vi "Read Exit Slit.vi"(8 "error in (no error)":errorcluster, 11 "Spectrometer Digikröm in":refnum<class "Spectrometer Digikröm.lvclass">) -> (0 "error out":errorcluster, 2 "Exit Slit":dbl[unit]=9.999999999999999e-06, 3 "Spectrometer Digikröm out":refnum<class "Spectrometer Digikröm.lvclass">)   [LabVIEW 2017, in "Spectrometer Digikröm.lvclass"]
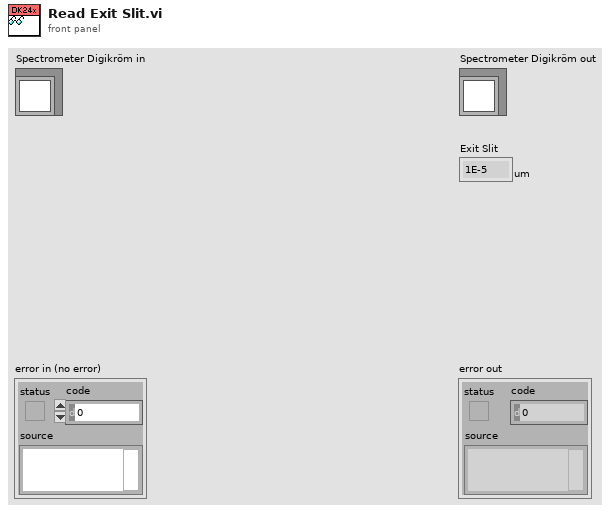
[diagram p1: front panel]
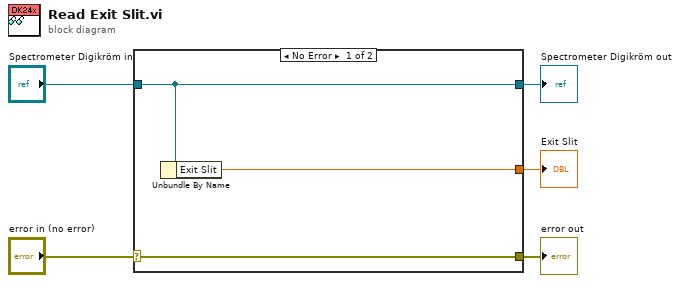
[diagram p0: block diagram]
diagram:
  n1 = case shown="No Error" "error in (no error)" {
    selector: "error in (no error)" -> [w8 w9]
    tunnel: [w8 w9] -> w4
    tunnel: [w7 w10] -> w2
    tunnel: "Spectrometer Digikröm in" -> [w7 w10]
    tunnel: [w6 _] -> w1
    frame No Error {
      n2 = Unbundle By Name(w7) -> ("Exit Slit"=w6:dbl[unit])
    }
    frame Error {
    }
  }
  "error out" <- w4
  "Spectrometer Digikröm out" <- w2
  "Exit Slit" <- w1
